vi "Load McP CounterPos.dat.V0.50.vi"(0 "McP Counter Position Path":path) -> (1 "Counter Position":dbl=1620.34567 format="%.5f", 2 "Stepper Position":i32, 3 "Last Calibration Date":string=" 1620.34567\r")   [LabVIEW 2025]
doc: "Author: Scott Hannahs <sth@magnet.fsu.edu>\n\nThis software is licensed for use under the “MIT License\"\nCopyright (c) 2025 Scott Hannahs, sth@sth@magnet.sthnet.net\n\nPermission is hereby granted, free of charge, to any person obtaining a copy of this software and associated documentation files (the \"Software\"), to deal in the Software without restriction, including without limitation the rights to use, copy, modify, merge, publish, distribute, sublicense, and/or sell copies of the Software, and to permit persons to whom the Software is furnished to do so, subject to the following conditions: The above copyright notice and this permission notice shall be included in all copies or substantial portions of the Software.\n\nTHE SOFTWARE IS PROVIDED \"AS IS\", WITHOUT WARRANTY OF ANY KIND, EXPRESS OR IMPLIED, INCLUDING BUT NOT LIMITED TO THE WARRANTIES OF MERCHANTABILITY, FITNESS FOR A PARTICULAR PURPOSE AND NONINFRINGEMENT. IN NO EVENT SHALL THE AUTHORS OR COPYRIGHT HOLDERS BE LIABLE FOR ANY CLAIM, DAMAGES OR OTHER LIABILITY, WHETHER IN AN ACTION OF CONTRACT, TORT OR OTHERWISE, ARISING FROM, OUT OF OR IN CONNECTION WITH THE SOFTWARE OR THE USE OR OTHER DEALINGS IN THE SOFTWARE."
panel:
  out "MCP Counter Position .dat path":path
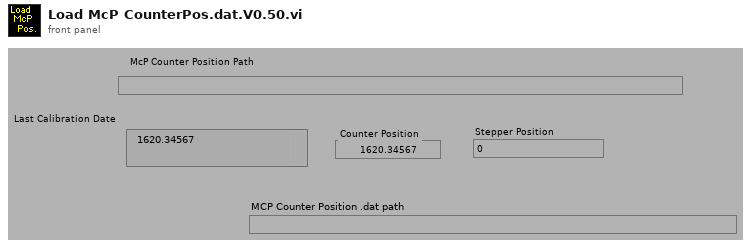
[diagram p1: front panel]
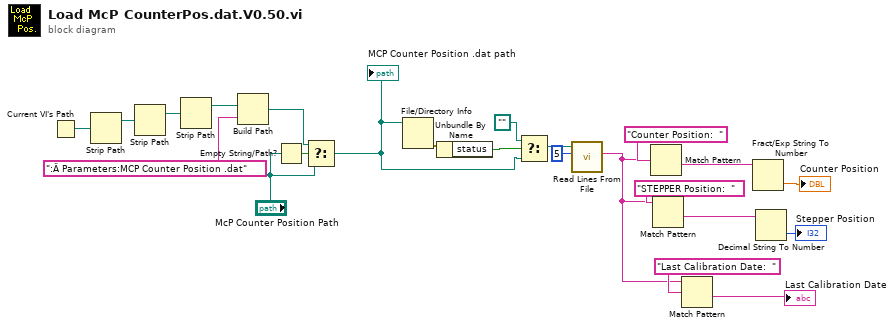
[diagram p0: block diagram]
diagram:
  n1 = Current VI's Path() -> (path=w3:path)
  n2 = Strip Path(path=w3) -> (stripped path=w8:path)  [unwired: 1 out]
  n3 = Strip Path(path=w8) -> (stripped path=w7:path)  [unwired: 1 out]
  n4 = Strip Path(path=w7) -> (stripped path=w4:path)  [unwired: 1 out]
  n5 = Build Path(base path=w4, name or relative path=":Ä Parameters:MCP Counter Position .dat") -> (appended path=w2:path)
  n6 = Empty String/Path?(string/path="McP Counter Position Path") -> (empty?=w9:bool)
  n7 = Select(t=w2, s=w9, f="McP Counter Position Path") -> (s? t:f=w1:path)
  "MCP Counter Position .dat path" <- w1
  n8 = File/Directory Info(path=w1) -> (error out=w13:errorcluster)  [unwired: 1 in, 6 out]
  n9 = Unbundle By Name(w13) -> ("status"=w12:bool)
  n10 = Select(t=path "", s=w12, f=w1) -> (s? t:f=w10:path)
  n11 = call <vilib>:"Read Lines From File.vi"("file path (dialog if empty)"=w10, "number of lines (all:-1)"=5) -> ("line string"=w15:string)  [unwired: 4 in, 3 out]
  n12 = Match Pattern(string=w15, regular expression="Counter Position:  ") -> (after substring=w17:string)  [unwired: 1 in, 3 out]
  n13 = Match Pattern(string=w15, regular expression="STEPPER Position:  ") -> (after substring=w14:string)  [unwired: 1 in, 3 out]
  n14 = Match Pattern(string=w15, regular expression="Last Calibration Date:  ") -> (after substring=→"Last Calibration Date":string)  [unwired: 1 in, 3 out]
  n15 = Fract/Exp String To Number(string=w17) -> (number=→"Counter Position":dbl)  [unwired: 3 in, 1 out]
  n16 = Decimal String To Number(string=w14) -> (number=→"Stepper Position":i32)  [unwired: 2 in, 1 out]
